vi "Test_API_DelayedShutdown_PostCloseLogAvailable.vi"(8 "error in (no error)":errorcluster, 11 "TestCase in":refnum<class "TestComposedLog.lvclass">) -> (0 "error out":errorcluster, 3 "TestCase out":refnum<class "TestComposedLog.lvclass">)   [LabVIEW 2017, in "TestComposedLog.lvclass"]
uses:
  TestComposedLog.lvclass
  Source/Composed Log/LoggerReference/LoggerReference.lvclass/LoggerReference.ctl
  b0748f28-e60e-4d9b-915d-00834a7f2ea6.vi
  b0748f28-e60e-4d9b-915d-00834a7f2ea6.vi/1a5055d8-93b4-4dff-95b8-2d840e1efea5.vi
  Source/Composed Log/LoggerReference/Return Aggregate Queues.vi
  Source/Composed Log/LoggerReference/Add Aggregate Log.vi
  b0748f28-e60e-4d9b-915d-00834a7f2ea6.vi/1a5055d8-93b4-4dff-95b8-2d840e1efea5.vi/552da71b-c3a6-4840-b515-a419b546c917.vi
  Source/Composed Log/LoggerReference/Log.vi
  Source/Composed Log/LoggerReference/Get Valid Event Time.vi
  Source/Composed Log/LoggerReference/Send Add Sink.vi
  Source/Composed Log/LoggerReference/Remove Stale Logs.vi
  Source/LVQueue Sink/LVQueue Sink.lvclass
  C:/CS/Internal/LabVIEW/Logger/Source/Composed Log/Log Sink/Log Sink.lvclass
  Source/Composed Log/Application Logger/Launch Worker Loop.vi
  Source/Composed Log/LoggerReference/Initialize Logger Instance.vi
  Source/Composed Log/Singleton Event Log/Logger Queue FGV.vi
  Source/Composed Log/IErrorFormat/IErrorFormat.lvclass
  Source/Composed Log/LoggerReference/LoggerReference.lvclass
  Source/Composed Log/Log Sink/Log Sink.lvclass
  <vilib>/addons/_JKI Toolkits/VI Tester/TestCase.llb/TestCase.lvclass
  Source/Composed Log/Singleton Event Log/Singleton Event Log.lvlib
  C:/Program Files (x86)/National Instruments/LabVIEW 2017/vi.lib/addons/_JKI Toolkits/VI Tester/TestCase.llb/TestCase.lvclass
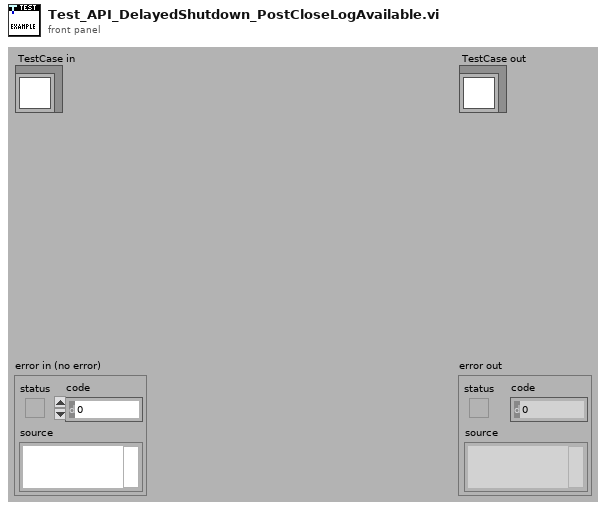
[diagram p1: front panel]
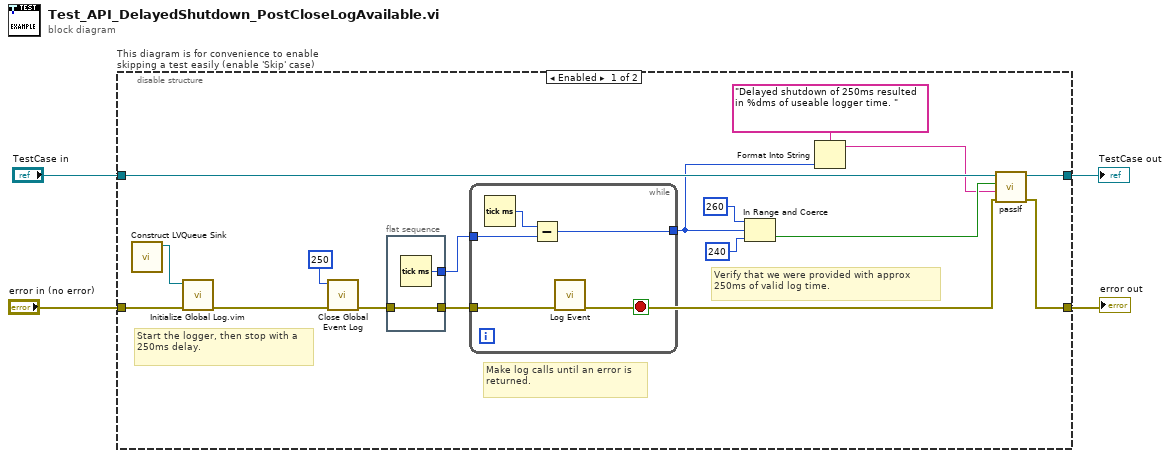
[diagram p0: block diagram]
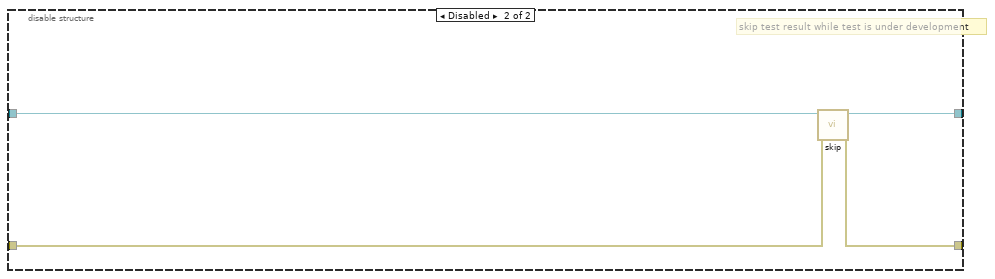
[diagram p2: hidden frame]
diagram:
  n1 = disable-structure "This diagram is for convenience to enable skipping a test easily (enable 'Skip' case)" shown="Enabled" {
    disable-tunnel: "TestCase in" -> [w16 w31]
    disable-tunnel: [w15 w29] -> w1
    disable-tunnel: [w14 w30] -> w3
    disable-tunnel: "error in (no error)" -> [w6 w28]
    frame Enabled {
      # "Verify that we were provided with approx 250ms of valid log time."
      # "Make log calls until an error is returned."
      # "Start the logger, then stop with a 250ms delay."
      n2 = call "Construct LVQueue Sink.vi"() -> ("LVQueue Sink out"=w5:refnum<class "LVQueue Sink.lvclass">)  [unwired: 10 in, 1 out]
      n3 = call "Initialize Global Log.vim"("error in (no error)"=w6, "Log Sink(s)"=w5) -> ("error out"=w20:errorcluster)  [unwired: 8 in, 1 out]
      n4 = call "Close Global Event Log.vi"("error in (no error)"=w20, "Deferred Close Time (0 ms)"=u32 250 ("Deferred Close Time (ms)")) -> ("error out"=w18:errorcluster)  [unwired: 9 in]
      n5 = flat-sequence {
        tunnel: w18 -> [w22]
        tunnel: [w22] -> w12
        tunnel: [w21] -> w17
        frame #0 {
          n6 = Tick Count (ms)() -> (millisecond timer value=w21:u32)
        }
      }
      n7 = while {
        tunnel: w12 -> [w24]
        tunnel: w17 -> [w26]
        tunnel: [w25] -> w10
        stop <- w23 stop-if-true
        n8 = Tick Count (ms)() -> (millisecond timer value=w27:u32)
        n9 = Subtract(x=w27, y=w26) -> (x-y=w25:u32)
        n10 = call "Log Event.vi"("error in (no error)"=w24) -> ("error out"=w23:errorcluster)  [unwired: 10 in]
      }
      n11 = In Range and Coerce(upper limit=u32 260 ("lower limit"), x=w10, lower limit=u32 240 ("upper limit")) -> (In Range?=w13:bool)  [unwired: 1 out]
      n12 = Format Into String(format string="Delayed shutdown of 250ms resulted in %dms of useable logger time. ", w10) -> (resulting string=w9:string)  [unwired: 2 in, 1 out]
      n13 = call-dynamic "passIf.vi"("error in (no error)"=w12, "message (\"\")"=w9, "pass"=w13, "TestCase in"=w16) -> ("error out"=w14:errorcluster, "TestCase out"=w15:refnum<class "TestComposedLog.lvclass">)  [unwired: 6 in]
    }
    frame Disabled {
      # "skip test result while test is under development"
      n14 = call <vilib>:"skip.vi"("error in (no error)"=w28, "TestCase in"=w31) -> ("error out"=w30:errorcluster, "TestCase out"=w29:refnum<class "TestComposedLog.lvclass">)  [unwired: 8 in]
    }
  }
  "error out" <- w3
  "TestCase out" <- w1
